vi "Get gRPC ID.vi"(11 "OOP Server in":refnum<class "server1.lvclass">) -> (2 "gRPC ID":T1, 3 "OOP Server out":refnum<class "server1.lvclass">)   [LabVIEW 2020, in "server1.lvlib" / "server1.lvclass"]
uses:
  server1.lvclass
  gRPC lvSupport/Server API/typeDefs/grpcId.ctl
  server1.lvclass/server1.ctl
  gRPC lvSupport/gprc-lvsupport.lvlib
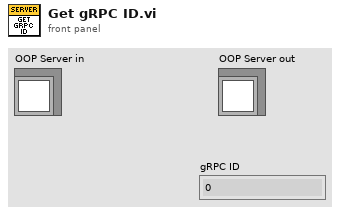
[diagram p1: front panel]
types:
  T1 = typedef "server1.lvlib/gprc-lvsupport.lvlib/grpcId.ctl" = u64
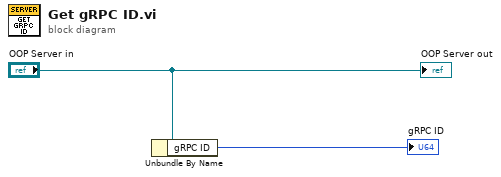
[diagram p0: block diagram]
diagram:
  n1 = Unbundle By Name("OOP Server in") -> ("gRPC ID"=→"gRPC ID":T1)
  "OOP Server out" <- "OOP Server in"
